vi "CreateToolbarObject.vi"(0 "reference in":refnum<class "DqmhModuleDiagramGraph.lvclass">, 2 "GraphButton":u32, 5 "error in (no error)":errorcluster) -> (14 "reference out":refnum<class "DqmhModuleDiagramGraph.lvclass">, 15 "toolType":T1, 16 "Edge":refnum<class "AbstractEdge.lvclass">, 17 "Node":refnum<class "AbstractNode.lvclass">, 18 "ButtonNameCompressed)":string, 19 "error out":errorcluster)   [LabVIEW 2020, in "DqmhModuleDiagramGraph.lvclass"]
uses:
  <resource>/Framework/Providers/Open_GDS/UML/DqmhModuleDiagramGraph_class/DqmhModuleDiagramGraph.lvclass
  <resource>/Framework/Providers/Open_GDS/UML/UMLEditor/UMLEditor tooltype.ctl
  <resource>/Framework/Providers/Open_GDS/UML/AbstractEdge_class/AbstractEdge.lvclass
  <resource>/Framework/Providers/Open_GDS/UML/AbstractNode_class/AbstractNode.lvclass
  <resource>/Framework/Providers/Open_GDS/UML/ArrowHead_class/ArrowHeadType.ctl
  <resource>/Framework/Providers/Open_GDS/UML/BentStyle_class/BentStyleType.ctl
  <resource>/Framework/Providers/Open_GDS/UML/LineStyle_class/LineStyleType.ctl
  <resource>/Framework/Providers/Open_GDS/UML/Graph_class/ToolbarButtonType.ctl
  <resource>/Framework/Providers/Open_GDS/UML/Graphics_class/StrokeType.ctl
  <resource>/Framework/Providers/Open_GDS/UML/VINode_class/VINode.lvclass
  C:/Program Files (x86)/National Instruments/LabVIEW 2020/resource/Framework/Providers/Open_GDS/UML/RectangularNode_class/RectangularNode.lvclass
  <resource>/Framework/Providers/Open_GDS/UML/DQMHModuleNode_class/DQMHModuleNode.lvclass
  <resource>/Framework/Providers/Open_GDS/UML/NoteNode_class/NoteNode.lvclass
  <resource>/Framework/Providers/Open_GDS/UML/ClassRelationshipEdge_class/ClassRelationshipEdge.lvclass
  C:/Program Files (x86)/National Instruments/LabVIEW 2020/resource/Framework/Providers/Open_GDS/UML/GeneralPathEdge_class/GeneralPathEdge.lvclass
  <resource>/Framework/Providers/Open_GDS/UML/NoteEdge_class/NoteEdge.lvclass
  <resource>/Framework/Providers/Open_GDS/UML/GeneralPathEdge_class/GeneralPathEdge.lvclass
  C:/Program Files (x86)/National Instruments/LabVIEW 2020/resource/Framework/Providers/Open_GDS/UML/AbstractEdge_class/AbstractEdge.lvclass
  <resource>/Framework/Providers/Open_GDS/UML/RectangularNode_class/RectangularNode.lvclass
  C:/Program Files (x86)/National Instruments/LabVIEW 2020/resource/Framework/Providers/Open_GDS/UML/AbstractNode_class/AbstractNode.lvclass
  <resource>/Framework/Providers/Open_GDS/UML/Graphics_class/Graphics.lvclass
  <resource>/Framework/Providers/Open_GDS/UML/ArrowHead_class/ArrowHead.lvclass
  <resource>/Framework/Providers/Open_GDS/UML/BentStyle_class/BentStyle.lvclass
  <resource>/Framework/Providers/Open_GDS/UML/LineStyle_class/LineStyle.lvclass
  <resource>/Framework/Providers/Open_GDS/UML/Graph_class/Graph.lvclass
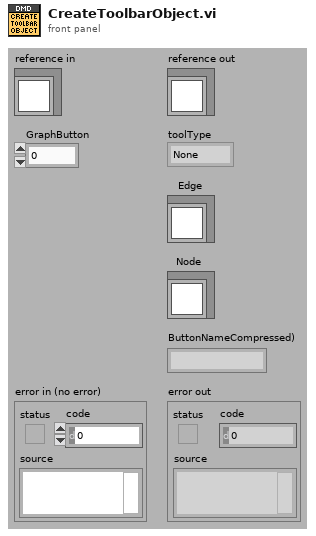
[diagram p1: front panel]
types:
  T1 = typedef "UMLEditor tooltype.ctl" = enum16{"None", "Node", "Edge"}
  T2 = typedef "Graph.lvclass/ToolbarButtonType.ctl" = cluster{"Text":string, "Type":T1}
  T3 = typedef "LineStyle.lvclass/LineStyleType.ctl" = enum16{"SOLID", "DOTTED"}
  T4 = typedef "BentStyle.lvclass/BentStyleType.ctl" = enum16{"STRAIGHT", "HV", "VH", "HVH", "VHV", "ARC"}
  T5 = typedef "ArrowHead.lvclass/ArrowHeadType.ctl" = enum16{"NONE", "TRIANGLE", "BLACK_TRIANGLE", "V", "HALF_V", "DIAMOND", "BLACK_DIAMOND"}
  T6 = typedef "Graphics.lvclass/StrokeType.ctl" = enum16{"USE_DEFAULT", "SOLID", "DOTTED"}
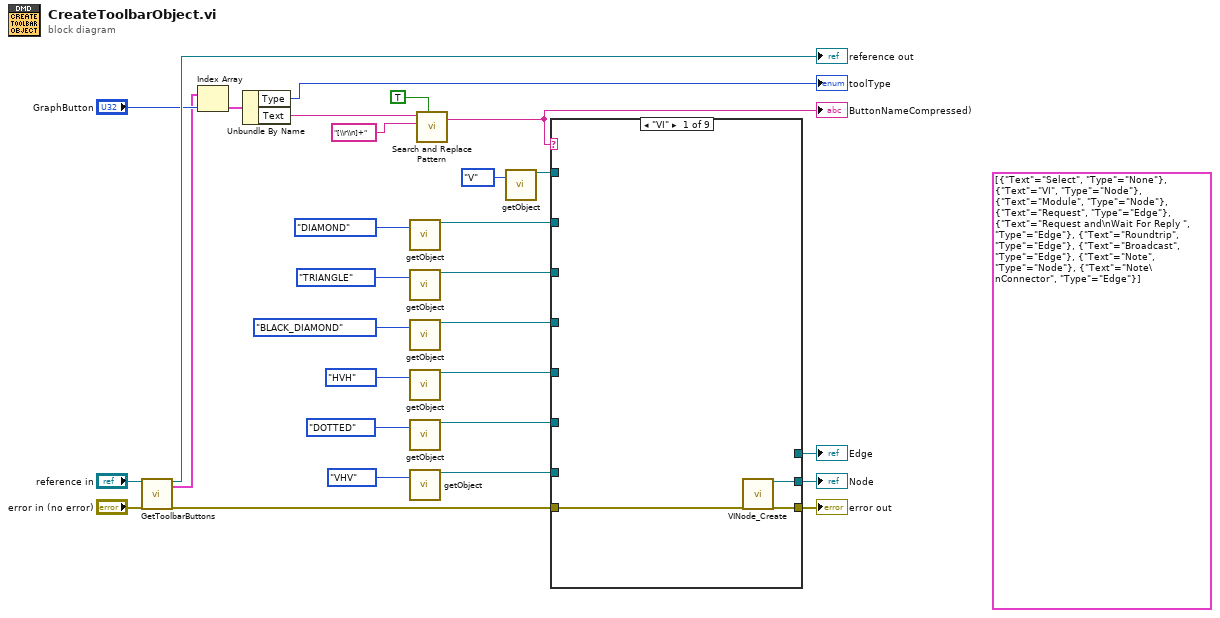
[diagram p0: block diagram]
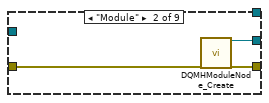
[diagram p2: hidden frame]
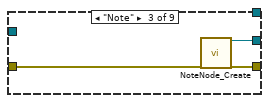
[diagram p3: hidden frame]
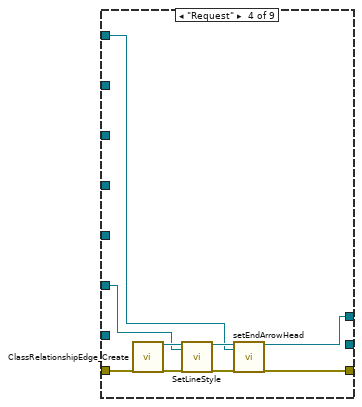
[diagram p4: hidden frame]
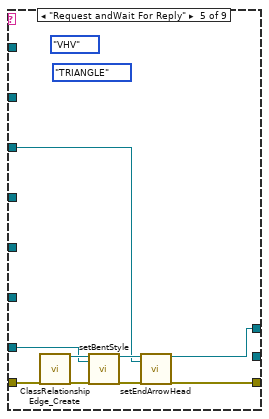
[diagram p5: hidden frame]
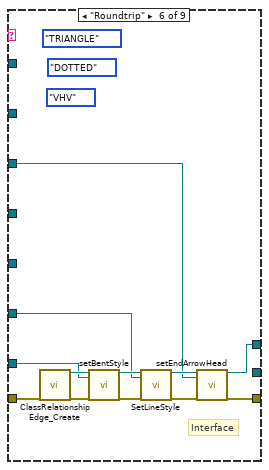
[diagram p6: hidden frame]
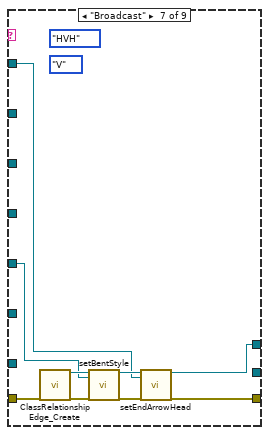
[diagram p7: hidden frame]
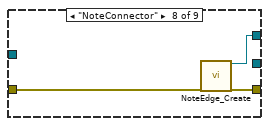
[diagram p8: hidden frame]
diagram:
  (unwired) T2[] [{"Text"="Select", "Type"=enum."None"}, {"Text"="VI", "Type"=enum."Node"}, {"Text"="Module", "Type"=enum."Node"}, {"Text"="Request", "Type"=enum."Edge"}, {"Text"="Request and\nWait For Reply ", "Type"=enum."Edge"}, {"Text"="Roundtrip", "Type"=enum."Edge"}, {"Text"="Broadcast", "Type"=enum."Edge"}, {"Text"="Note", "Type"=enum."Node"}, {"Text"="Note\nConnector", "Type"=enum."Edge"}] ("ToolbarButtons")
  n1 = call-dynamic "GetToolbarButtons.vi"("reference in"="reference in", "error in (no error)"="error in (no error)") -> ("reference out"=→"reference out":refnum<class "DqmhModuleDiagramGraph.lvclass">, "ToolbarButtons"=w20:T2[], "error out"=w11:errorcluster)  [unwired: 13 in, 2 out]
  n2 = Index Array(array=w20, index="GraphButton") -> (element=w19:T2)
  n3 = Unbundle By Name(w19) -> ("Type"=→"toolType":T1, "Text"=w3:string)
  n4 = call <resource>:"getObject.vi"("arrowHead"=ArrowHeadType."DIAMOND") -> ("reference out"=w5:refnum<class "ArrowHead.lvclass">)  [unwired: 1 in, 17 out]
  n5 = call <resource>:"getObject.vi"("arrowHead"=ArrowHeadType."TRIANGLE") -> ("reference out"=w7:refnum<class "ArrowHead.lvclass">)  [unwired: 1 in, 17 out]
  n6 = call <resource>:"getObject.vi"("arrowHead"=ArrowHeadType."BLACK_DIAMOND") -> ("reference out"=w4:refnum<class "ArrowHead.lvclass">)  [unwired: 1 in, 17 out]
  n7 = call <resource>:"getObject.vi"("bentStyle"=BentStyleType."HVH") -> ("reference out"=w6:refnum<class "BentStyle.lvclass">)  [unwired: 1 in, 17 out]
  n8 = call <resource>:"getObject.vi"("lineStyle"=LineStyleType."DOTTED") -> ("reference out"=w10:refnum<class "LineStyle.lvclass">)  [unwired: 1 in, 17 out]
  n9 = call <resource>:"getObject.vi"("bentStyle"=BentStyleType."VHV") -> ("reference out"=w8:refnum<class "BentStyle.lvclass">)  [unwired: 1 in, 17 out]
  n10 = call <vilib>:"Search and Replace Pattern.vi"("string"=w3, "regular expression (\"\")"="[\\r\\n]+" ("regular expression (\"\")"), "replace all? (F)"=TRUE) -> ("result string"=w21:string)  [unwired: 2 in, 1 out]
  "ButtonNameCompressed)" <- w21
  n11 = call <resource>:"getObject.vi"("arrowHead"=ArrowHeadType."V") -> ("reference out"=w9:refnum<class "ArrowHead.lvclass">)  [unwired: 1 in, 17 out]
  n12 = case shown="\"VI\"" w21 {
    tunnel: w11 -> [w32 w35 w38 w45 w54 w62 w73 w80 w81]
    tunnel: [w31 w34 w37 w42 w51 w61 w72 w79 w81] -> w28
    tunnel: [w30 w33 w36 _ _ _ _ _ _] -> w23
    tunnel: w10 -> [_ _ _ w41 _ w59 _ _ _]
    tunnel: w9 -> [_ _ _ w40 _ _ w70 _ _]
    tunnel: w8 -> [_ _ _ _ w50 w60 _ _ _]
    tunnel: w7 -> [_ _ _ _ w49 w58 _ _ _]
    tunnel: w6 -> [_ _ _ _ _ _ w71 _ _]
    tunnel: w5 -> [_ _ _ _ _ _ _ _ _]
    tunnel: w4 -> [_ _ _ _ _ _ _ _ _]
    tunnel: [_ _ _ w39 w48 w57 w69 w78 _] -> w22
    frame "VI" {
      n13 = call <resource>:"VINode_Create.vi"("error in (no error)"=w32) -> ("reference out"=w30:refnum<class "VINode.lvclass">, "error out"=w31:errorcluster)  [unwired: 17 in]
    }
    frame "Module" {
      n14 = call <resource>:"DQMHModuleNode_Create.vi"("error in (no error)"=w35) -> ("reference out"=w33:refnum<class "DQMHModuleNode.lvclass">, "error out"=w34:errorcluster)  [unwired: 17 in]
    }
    frame "Note" {
      n15 = call <resource>:"NoteNode_Create.vi"("error in (no error)"=w38) -> ("reference out"=w36:refnum<class "NoteNode.lvclass">, "error out"=w37:errorcluster)  [unwired: 1 in, 16 out]
    }
    frame "Request" {
      n16 = call <resource>:"ClassRelationshipEdge_Create.vi"("error in (no error)"=w45) -> ("reference out"=w46:refnum<class "ClassRelationshipEdge.lvclass">, "error out"=w44:errorcluster)  [unwired: 1 in, 16 out]
      n17 = call-dynamic "SetLineStyle.vi"("reference"=w46, "lineStyle"=w41, "error in (no error)"=w44) -> ("reference out"=w47:refnum<class "ClassRelationshipEdge.lvclass">, "error out"=w43:errorcluster)  [unwired: 15 in]
      n18 = call-dynamic "setEndArrowHead.vi"("reference"=w47, "endArrowHead"=w40, "error in (no error)"=w43) -> ("reference out"=w39:refnum<class "ClassRelationshipEdge.lvclass">, "error out"=w42:errorcluster)  [unwired: 15 in]
    }
    frame "Request andWait For Reply" {
      (unwired) BentStyleType."VHV" ("bentStyle")
      (unwired) ArrowHeadType."TRIANGLE" ("arrowHead")
      n19 = call <resource>:"ClassRelationshipEdge_Create.vi"("error in (no error)"=w54) -> ("reference out"=w56:refnum<class "ClassRelationshipEdge.lvclass">, "error out"=w53:errorcluster)  [unwired: 1 in, 16 out]
      n20 = call <resource>:"setBentStyle.vi"("reference"=w56, "newBentStyle"=w50, "error in (no error)"=w53) -> ("reference out"=w55:refnum<class "ClassRelationshipEdge.lvclass">, "error out"=w52:errorcluster)  [unwired: 15 out]
      n21 = call-dynamic "setEndArrowHead.vi"("reference"=w55, "endArrowHead"=w49, "error in (no error)"=w52) -> ("reference out"=w48:refnum<class "ClassRelationshipEdge.lvclass">, "error out"=w51:errorcluster)  [unwired: 15 in]
    }
    frame "Roundtrip" {
      (unwired) StrokeType."DOTTED" ("lineStyle")
      (unwired) BentStyleType."VHV" ("bentStyle")
      (unwired) ArrowHeadType."TRIANGLE" ("arrowHead")
      # "Interface"
      n22 = call <resource>:"ClassRelationshipEdge_Create.vi"("error in (no error)"=w62) -> ("reference out"=w63:refnum<class "ClassRelationshipEdge.lvclass">, "error out"=w64:errorcluster)  [unwired: 1 in, 16 out]
      n23 = call <resource>:"setBentStyle.vi"("reference"=w63, "newBentStyle"=w60, "error in (no error)"=w64) -> ("reference out"=w65:refnum<class "ClassRelationshipEdge.lvclass">, "error out"=w66:errorcluster)  [unwired: 15 out]
      n24 = call-dynamic "SetLineStyle.vi"("reference"=w65, "lineStyle"=w59, "error in (no error)"=w66) -> ("reference out"=w67:refnum<class "ClassRelationshipEdge.lvclass">, "error out"=w68:errorcluster)  [unwired: 15 in]
      n25 = call-dynamic "setEndArrowHead.vi"("reference"=w67, "endArrowHead"=w58, "error in (no error)"=w68) -> ("reference out"=w57:refnum<class "ClassRelationshipEdge.lvclass">, "error out"=w61:errorcluster)  [unwired: 15 in]
    }
    frame "Broadcast" {
      (unwired) BentStyleType."HVH" ("bentStyle")
      (unwired) ArrowHeadType."V" ("arrowHead")
      n26 = call <resource>:"ClassRelationshipEdge_Create.vi"("error in (no error)"=w73) -> ("reference out"=w74:refnum<class "ClassRelationshipEdge.lvclass">, "error out"=w75:errorcluster)  [unwired: 1 in, 16 out]
      n27 = call <resource>:"setBentStyle.vi"("reference"=w74, "newBentStyle"=w71, "error in (no error)"=w75) -> ("reference out"=w76:refnum<class "ClassRelationshipEdge.lvclass">, "error out"=w77:errorcluster)  [unwired: 15 out]
      n28 = call-dynamic "setEndArrowHead.vi"("reference"=w76, "endArrowHead"=w70, "error in (no error)"=w77) -> ("reference out"=w69:refnum<class "ClassRelationshipEdge.lvclass">, "error out"=w72:errorcluster)  [unwired: 15 in]
    }
    frame "NoteConnector" {
      n29 = call <resource>:"NoteEdge_Create.vi"("error in (no error)"=w80) -> ("reference out"=w78:refnum<class "NoteEdge.lvclass">, "error out"=w79:errorcluster)  [unwired: 1 in, 16 out]
    }
    frame "Select", Default {
    }
  }
  "error out" <- w28
  "Edge" <- w22
  "Node" <- w23
